vi "PlotSettings.vi"(2 "Detectorin":u32=1, 3 "Sourcein":u32=1) -> (0 "Detector#":u32=1, 1 "Source#":u32=1)   [LabVIEW 2016]
doc: "Source-Detector number input for Flow Plot"
panel:
  in  "Cancel":bool
  in  "Apply":bool
  in  "Detector Number:":string(combo)="1"
  in  "Source Number:":string(combo)="1"
  # "Please Selelct Source-Detector Pair for Flow Plot"
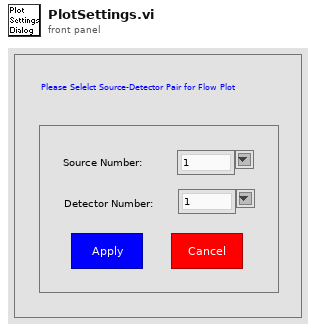
[diagram p1: front panel]
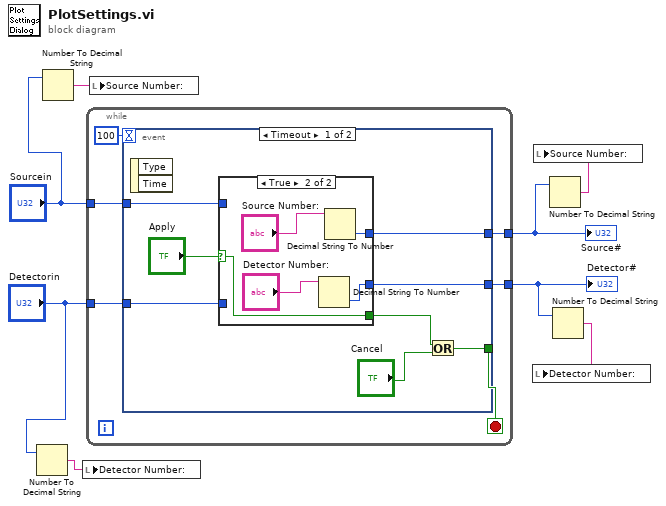
[diagram p0: block diagram]
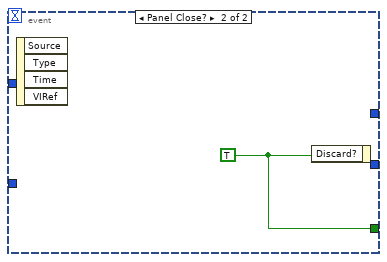
[diagram p3: hidden frame]
diagram:
  n1 = Number To Decimal String(number="Detectorin") -> (decimal integer string=w4:string)  [unwired: 1 in]
  n2 = Number To Decimal String(number="Sourcein") -> (decimal integer string=w3:string)  [unwired: 1 in]
  n3 = local write "Detector Number:"(w4) -> ()
  n4 = while {
    tunnel: [w13] -> w5
    tunnel: [w12] -> w6
    tunnel: "Sourcein" -> [w11]
    tunnel: "Detectorin" -> [w10]
    stop <- w14 stop-if-true
    n5 = event shown="[0] Timeout" {
      selector: _ -> [_ _]
      dyn-events: _ -> [_ _]
      timeout: 100 -> [_ _]
      tunnel: [w19 w30] -> w14
      tunnel: [w16 _] -> w13
      tunnel: [w15 _] -> w12
      tunnel: w11 -> [w18 _]
      tunnel: w10 -> [w17 _]
      event Timeout {
        n6 = event-data() -> ()  [unwired: 1 in, 2 out]
        n7 = case shown="True" "Apply" {
          selector: "Apply" -> [_ w27]
          tunnel: [_ w27] -> w21
          tunnel: [w24 w28] -> w16
          tunnel: [w23 w26] -> w15
          tunnel: w18 -> [w24 _]
          tunnel: w17 -> [w23 _]
          frame False {
          }
          frame True {
            n8 = Decimal String To Number(string="Detector Number:") -> (number=w26:i32)  [unwired: 2 in, 1 out]
            n9 = Decimal String To Number(string="Source Number:") -> (number=w28:i32)  [unwired: 2 in, 1 out]
          }
        }
        n10 = Or(x=w21, y="Cancel") -> (x .or. y?=w19:bool)
      }
      event Panel Close? {
        w30 = TRUE
        n11 = event-data() -> ()  [unwired: 1 in, 4 out]
        n12 = event-data("Discard?"=w30) -> ()  [unwired: 1 in, 1 out]
      }
    }
  }
  "Source#" <- w5
  "Detector#" <- w6
  n13 = local write "Source Number:"(w3) -> ()
  n14 = Number To Decimal String(number=w5) -> (decimal integer string=w8:string)  [unwired: 1 in]
  n15 = local write "Source Number:"(w8) -> ()
  n16 = Number To Decimal String(number=w6) -> (decimal integer string=w7:string)  [unwired: 1 in]
  n17 = local write "Detector Number:"(w7) -> ()
